vi "2022-TestCodeOnWindows.vi"() -> ()   [LabVIEW 2020]
panel:
  in  "error in":errorcluster
  out "error out":errorcluster
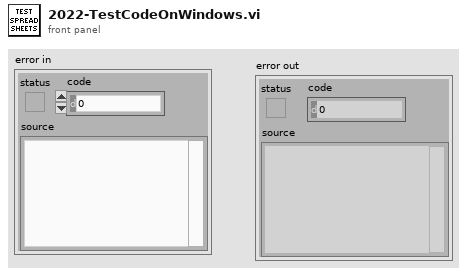
[diagram p1: front panel]
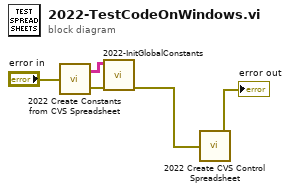
[diagram p0: block diagram]
diagram:
  n1 = call "2022 Create Constants from CVS Spreadsheet.vi"("error in"="error in") -> ("localConstantSpreadSheet"=w4:string[][], "error out"=w3:errorcluster)
  n2 = call "2022-InitGlobalConstants.vi"("error in (no error)"=w3, "localConstantSpreadSheet"=w4) -> ("error out"=w2:errorcluster)  [unwired: 9 in]
  n3 = call "2022 Create CVS Control Spreadsheet.vi"("error in"=w2) -> ("error out"=→"error out":errorcluster)
